vi "deleteData.vi"(8 "error in":errorcluster, 11 "SQL query":string="select * from t_area;") -> (0 "error out":errorcluster)   [LabVIEW 2014, in "DataBase.lvlib"]
uses:
  <vilib>/addons/database/Connection.llb/DB Tools Open Connec (String).vi
  <vilib>/addons/database/Connection.llb/Conn Execute.vi
  <vilib>/addons/database/Recordset.llb/Rec Destroy - Connection.vi
  DataBase.lvlib
  <vilib>/addons/database/NI_Database_API.lvlib
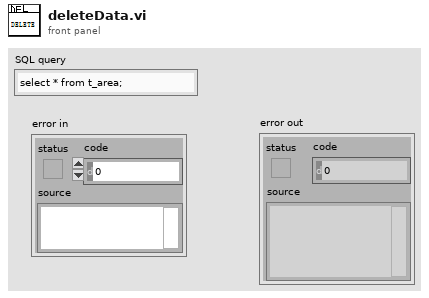
[diagram p1: front panel]
types:
  T1 = typedef "NI_Database_API.lvlib/Conn ObjectReference.ctl" = refnum<k1>
  T2 = typedef "NI_Database_API.lvlib/Rec ObjectReference.ctl" = refnum<k1>
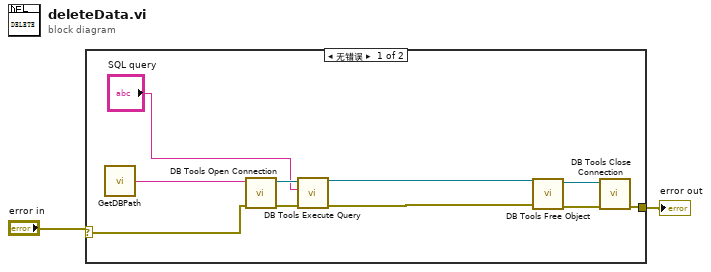
[diagram p0: block diagram]
diagram:
  n1 = case shown="无错误" "error in" {
    selector: "error in" -> [w8 w13]
    tunnel: [w7 w13] -> w1
    frame No Error {
      n2 = call "GetDBPath.vi"() -> ("Connection"=w6:string)  [unwired: 1 in]
      n3 = call-poly <vilib>:"DB Tools Open Connection.vi"("error in (no error)"=w8, "connection information"=w6) -> ("error out"=w11:errorcluster, "connection reference"=w12:T1)  [unwired: 6 in]
      n4 = call-poly <vilib>:"DB Tools Execute Query.vi"("error in (no error)"=w11, "SQL query"="SQL query", "connection reference"=w12) -> ("error out"=w3:errorcluster, "recordset reference"=w4:T2)  [unwired: 5 in]
      n5 = call-poly <vilib>:"DB Tools Free Object.vi"("error in (no error)"=w3, "recordset reference"=w4) -> ("error out"=w10:errorcluster, "connection reference"=w9:T1)  [unwired: 8 in]
      n6 = call <vilib>:"DB Tools Close Connection.vi"("error in (no error)"=w10, "connection reference"=w9) -> ("error out"=w7:errorcluster)  [unwired: 5 in]
    }
    frame Error {
    }
  }
  "error out" <- w1
